vi "Data_folder_Path.vi"(1 "seconds":dbl, 2 "Data Type":string="Colour Calib") -> (0 "Data Folder":path)   [LabVIEW 2010]
uses:
  Globals/Constants_global.vi
  Globals/Preference_global.vi
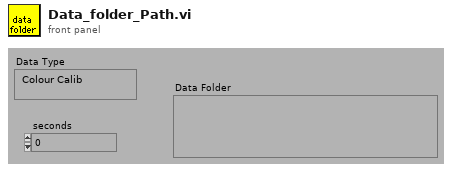
[diagram p1: front panel]
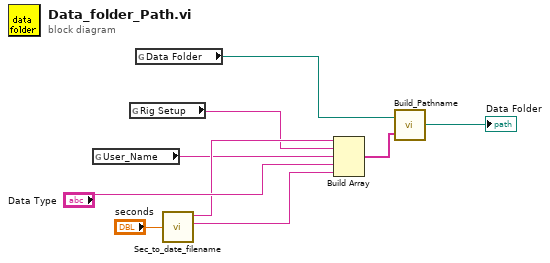
[diagram p0: block diagram]
diagram:
  n1 = global read "Preference_global.vi" "User_Name"() -> (w4:string)
  n2 = global read "Preference_global.vi" "Rig Setup"() -> (w3:string)
  n3 = global read "Constants_global.vi" "Data Folder"() -> (w6:path)
  n4 = call "Sec_to_date_filename.vi"("seconds"="seconds") -> ("Year"=w5:string, "Month"=w8:string)  [unwired: 2 out]
  n5 = Build Array(w5, w3, w4, "Data Type", w8) -> (w7:string[])
  n6 = call "Build_Pathname.vi"("Output Array"=w7, "Pathname"=w6) -> ("Appended path"=→"Data Folder":path)
